vi "fpga_sysID_Z_axis_simple.vi"() -> ()   [LabVIEW 2017]
uses:
  controls/boolean_info.ctl
  sysID_Z-axis-params.ctl
  <vilib>/rvi/Emulation/niFpgaGetClockAttributes.vi
  <vilib>/rvi/Emulation/niFpgaSctlEmulationGetInTimedLoop.vi
  <vilib>/rvi/Emulation/niFpgaEmulationReportErrorSimple.vi
  <vilib>/rvi/Emulation/niFpgaProcessEmulError.vi
  <vilib>/rvi/eio/common/nirviEmuTemplateMethod_errors.vi
  <vilib>/rvi/DataTransferAndStorage/Container/Common/niFpgaContainerExecOnDevCompGetState.vi
  <vilib>/rvi/Emulation/niFpgaEmulationIsFPGAContextNoSignature.vi
  <vilib>/rvi/errors/niFpgaSetErrorForExecOnDevCompSimple.vi
  <vilib>/rvi/eio/common/nirviEmuReportErrorAndStop.vi
  <vilib>/rvi/DataTransferAndStorage/Container/Common/niFpgaContainerGetUniqueNameForEmu.vi
  <vilib>/rvi/FIFO/Fifo_Resource/nirvififoEmulationSetSize.vi
  <vilib>/rvi/FIFO/Fifo_Resource/nirviFifoEmulationQueueMgr.vi
  <instcachedir>/0/nirviFifoEmulationQueueMgr_E5CAEC123FF24DC58D834DCA3CDAA9B5.lvgen/nirviFifoEmulationQueueMgr_E5CAEC123FF24DC58D834DCA3CDAA9B5_006.vi
  <vilib>/rvi/FIFO/Fifo_Resource/nirvififoEmulationDetermineInputValidOut.vi
  <vilib>/rvi/FIFO/Fifo_Resource/nirvififoEmulationCreateLock.vi
  <vilib>/rvi/FIFO/Fifo_Resource/nirvififoEmulationObtainLock.vi
  <vilib>/rvi/FIFO/Fifo_Resource/nirvififoEmulationReleaseLock.vi
  <vilib>/rvi/occurrence/nirviWaitOnOccurrenceBase.vi
  <vilib>/rvi/errors/nirviReportUnexpectedCaseInternalError.vi
  <vilib>/rvi/errors/nirviReportUnexpectedCaseInternalError (U32).vi
  <vilib>/Utility/error.llb/Clear Errors.vi
  <vilib>/rvi/interface/RandomDataEmulation/niFpgaRandomDataHandleErrors.vi
  <vilib>/rvi/Memory/Memory_Emulation/niFpgaMemoryEmulationCacheClearOnFirstRun.vi
  <vilib>/rvi/Memory/Memory_Emulation/nirvimemoryEmulationManagerCache_MakeExclusive.vi
  <vilib>/rvi/Memory/Memory_Emulation/niFpgaMemoryEmulationValidateCache.vi
  <vilib>/rvi/Memory/Memory_Emulation/nirvimemoryEmulationManagerCache_InsertValue.vi
  <vilib>/rvi/Memory/Memory_Emulation/nirvimemoryEmulationManagerCache_ReleaseExclusive.vi
  <vilib>/rvi/Memory/Memory_Emulation/nirvimemoryEmulationManagerCache_GetValue.vi
  <vilib>/rvi/Memory/Memory_Emulation/nirvimemoryEmulationManagerCache_SetValue.vi
  <vilib>/rvi/Emulation/niFpgaCriticalErrorInLSC.vi
  <vilib>/eio/EIONode/EIONode.xnode
  <vilib>/rvi/DataTransferAndStorage/Container/XNode/niFpgaContainer.xnode
  <vilib>/rvi/FIFO/Fifo_Resource/niFpgaFifoEmulationRefIn.vi
  <vilib>/rvi/DataTransferAndStorage/Register/Emulation/niFpgaRegisterEmulation.vi
  libimaging-cs.lvlib
panel:
  out "logging-timeout?":bool
  in  "sysID_Z_axis_params":T1={"TOL"=0.3, "ramp-rate"=-5e-06, "z-u-max"=5.0, "offset"=0.0, "Ki"=0.001, "Z-error-threshold"=0.0, "Z-settled-samples\nthreshold "=0, "z_UP"=1.5, "zup-N"=5000} {"Z-error-threshold" format="%#_13g"; "ramp-rate" format="%#_4g"; "TOL" format="%#_13g"}
  out "iter":i32
  out "All Done":bool
  in  "TsTicks":u32=1600
  out "Current Case":i16
  out "boolean \nindicators":T2
  out "z-u(k)":sgl
  in  "ABORT":bool
  out "read fifo HARD timeout":bool
  out "e(0) (threshhold init)":fxp<+/-,16,5>
  in  "init Z up":fxp<+/-,16,5>
  in  "trigger-0":bool
  in  "initial case":i16
  # "- If collect all = fasle and collect move = false,\nwe only collect measurement data.\n- If collect all = false, and collect move = true,\nwe collect measurement and move data.\n- If collect all = true, we collect everything."
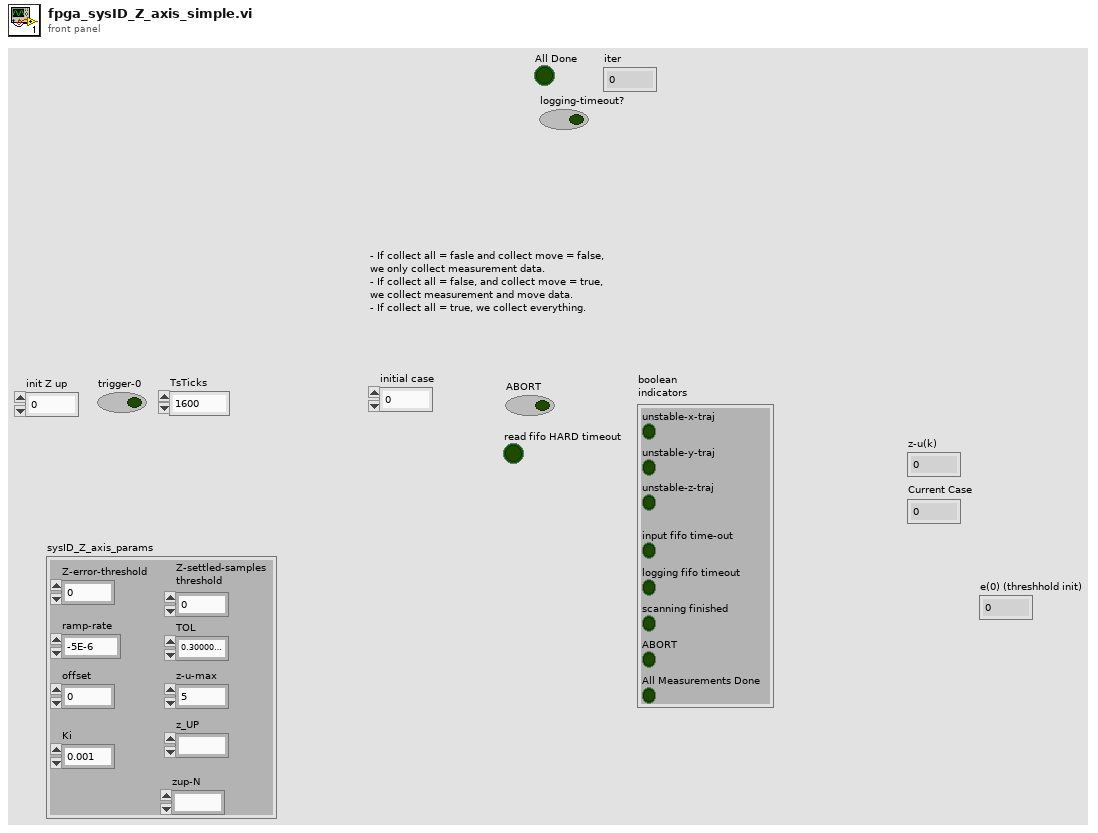
[diagram p1: front panel]
types:
  T1 = typedef "sysID_Z-axis-params.ctl" = cluster{"TOL":sgl, "ramp-rate":sgl, "z-u-max":sgl, "offset":sgl, "Ki":sgl, "Z-error-threshold":sgl, "Z-settled-samples\nthreshold ":i16, "z_UP":fxp<+/-,16,5>, "zup-N":i16}
  T2 = typedef "boolean_info.ctl" = cluster{"unstable-z-traj":bool, "input fifo time-out":bool, "logging fifo timeout":bool, "scanning finished":bool, "unstable-x-traj":bool, "unstable-y-traj":bool, "ABORT":bool, "All Measurements Done":bool}
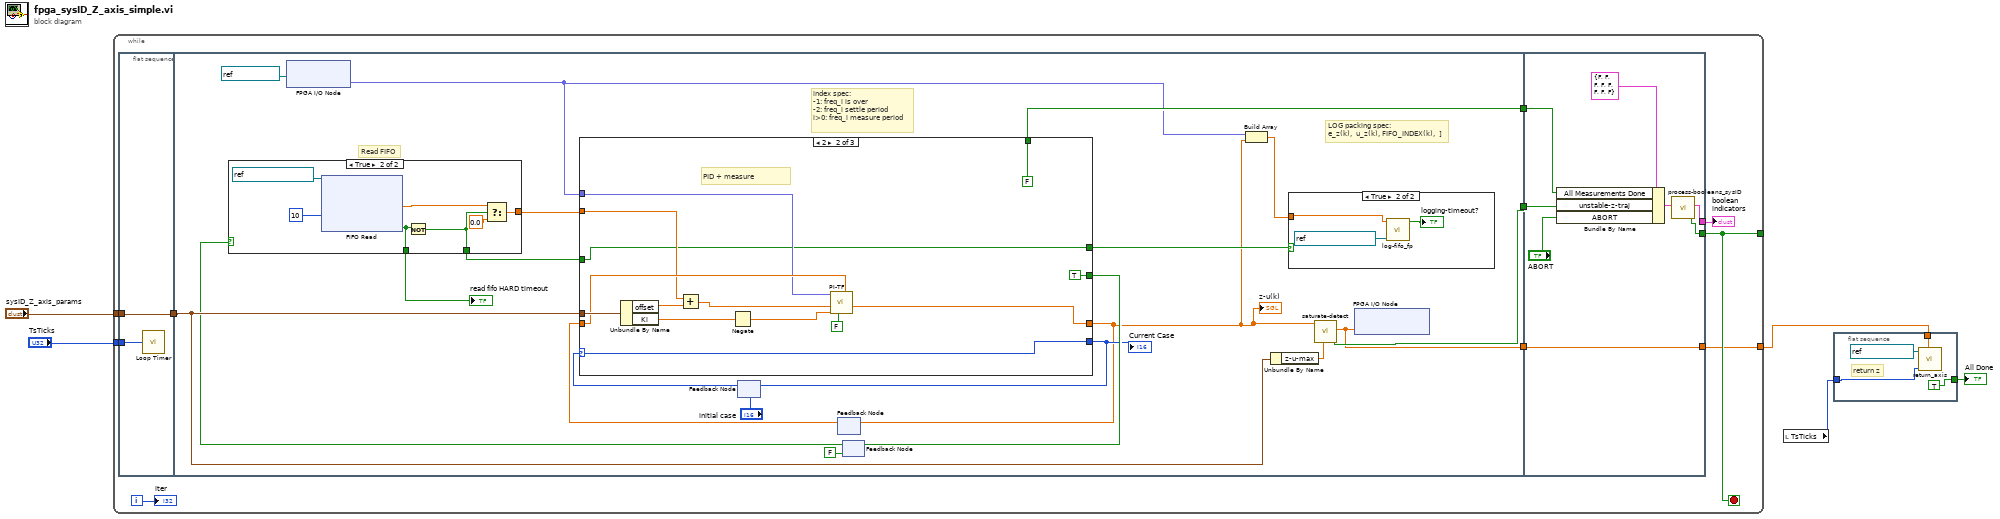
[diagram p0: block diagram]
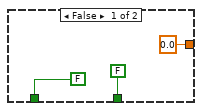
[diagram p3: hidden frame]
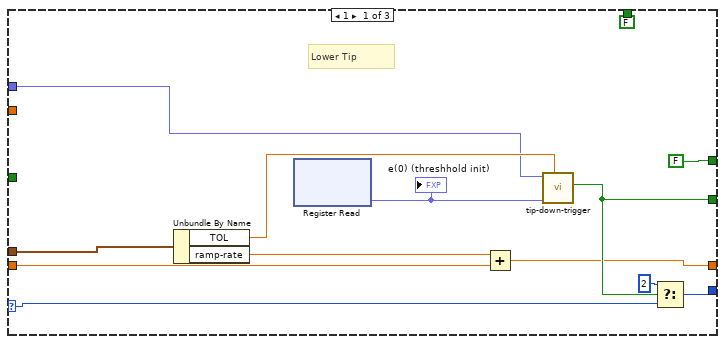
[diagram p4: hidden frame]
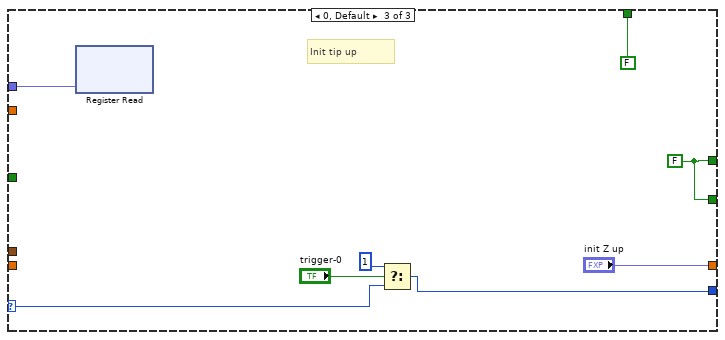
[diagram p5: hidden frame]
diagram:
  n1 = while {
    tunnel: "sysID_Z_axis_params" -> [w12]
    tunnel: "TsTicks" -> [w11]
    tunnel: [w9] -> _
    tunnel: [w7] -> w4
    i -> [w6]
    stop <- w9 stop-if-true
    n2 = flat-sequence {
      tunnel: w11 -> [w16]
      tunnel: w12 -> [w17]
      tunnel: [w17] -> w15
      tunnel: w15 -> [w29]
      tunnel: [w33] -> w14
      tunnel: [w27] -> w13
      tunnel: [w31] -> w8
      tunnel: w14 -> [w93]
      tunnel: w13 -> [w90]
      tunnel: [w86] -> w9
      tunnel: [w87] -> w10
      tunnel: [w89] -> w7
      tunnel: w8 -> [w89]
      frame #0 {
        n3 = call "Loop Timer"("Count(Ticks)"=w16) -> ()  [unwired: 1 out]
      }
      frame #1 {
        # "index spec:\n-1: freq_i is over\n-2: freq_i settle period\ni>0: freq_i measure period"
        # "LOG packing spec:\ne_z(k),  u_z(k), FIFO_INDEX(k),  ]"
        # "Read FIFO"
        n4 = xnode "FPGA I/O Node"("FPGA I/O In"=refnum<k21> "Mod2/AI2" ("y - ADC")) -> ("I/O Item"=w23:fxp<+/-,24,5>)  [unwired: 1 out]
        n5 = feedback #1("initial case") -> (w36:i16)
        n6 = feedback #2() -> (w35:sgl)  [unwired: 1 in]
        n7 = feedback #3(FALSE ("trigger-0")) -> (w18:bool)
        n8 = case shown="True" w18 {
          tunnel: [sgl 0.0 ("Element") w49] -> w30
          tunnel: [FALSE ("Timed Out?") w45] -> w21
          tunnel: [FALSE w44] -> w20
          frame False {
          }
          frame True {
            n9 = xnode ("FIFO Read")("Timeout"=10, "FIFO In"=refnum<k21> "host_to_fpga_fp") -> ("Element"=w46:sgl, "Timed Out?"=w45:bool)  [unwired: 1 out]
            n10 = Not(x=w45) -> (.not. x?=w44:bool)
            n11 = Select(t=w46, s=w44, f=sgl 0.0) -> (s? t:f=w49:sgl)
          }
        }
        "read fifo HARD timeout" <- w21
        n12 = case shown="2" w36 {
          selector: w36 -> [w60 w66 w83]
          tunnel: [FALSE w65 w78] -> w25
          tunnel: [w58 w66 w85] -> w26
          tunnel: w23 -> [w51 w68 w79]
          tunnel: [w53 TRUE ("trigger-0") w78] -> w32
          tunnel: [w52 w72 "init Z up"] -> w22
          tunnel: w35 -> [w56 w73 _]
          tunnel: w29 -> [w59 w74 _]
          tunnel: w30 -> [_ w67 _]
          tunnel: [FALSE FALSE FALSE] -> w27
          tunnel: w20 -> [_ w65 _]
          frame 1 {
            # "Lower Tip"
            n13 = Unbundle By Name(w59) -> ("TOL"=w62:sgl, "ramp-rate"=w61:sgl)
            n14 = xnode ("Register Read")() -> ("Data"=w63:fxp<+/-,16,5>)  [unwired: 1 in, 1 out]
            "e(0) (threshhold init)" <- w63
            n15 = Add(x=w61, y=w56) -> (x+y=w52:sgl)
            n16 = call "tip-down-trigger.vi"("TOL"=w62, "Vo"=w63, "e(k)"=w51) -> ("trigger"=w53:bool)  [unwired: 8 in]
            n17 = Select(t=i16 2, s=w53, f=w60) -> (s? t:f=w58:i16)
          }
          frame 2 {
            # "PID + measure"
            n18 = Unbundle By Name(w74) -> ("offset"=w70:sgl, "Ki"=w75:sgl)
            n19 = Add(x=w67, y=w70) -> (x+y=w71:sgl)
            n20 = Negate(x=w75) -> (-x=w76:sgl)
            n21 = call "PI-TF.vi"("u(k-1)"=w73, "reset"=FALSE, "Ki"=w76, "setpoint"=w71, "y(k)"=w68) -> ("u(k)"=w72:sgl)  [unwired: 6 in]
          }
          frame 0, Default {
            w78 = FALSE
            # "Init tip up"
            n22 = xnode ("Register Read")("Data"=w79) -> ()  [unwired: 1 in, 1 out]
            n23 = Select(t=i16 1, s="trigger-0", f=w83) -> (s? t:f=w85:i16)
          }
        }
        "z-u(k)" <- w22
        "Current Case" <- w26
        n24 = feedback-in #1(w26) -> ()
        n25 = feedback-in #2(w22) -> ()
        n26 = feedback-in #3(w32) -> ()
        n27 = Build Array(w23, w22) -> (w34:sgl[])
        n28 = Unbundle By Name(w29) -> ("z-u-max"=w28:sgl)
        n29 = case shown="True" w25 {
          tunnel: w34 -> [_ w40]
          frame False {
          }
          frame True {
            n30 = call "log-fifo_fp.vi"("FIFO In"=refnum<k21> "fpga_to_host_fp", "input-data"=w40) -> ("logging-timeout?"=→"logging-timeout?":bool)  [unwired: 9 in]
          }
        }
        n31 = call "saturate-detect.vi"("bound"=w28, "x"=w22) -> ("saturated"=w33:bool, "sat(x)"=w31:sgl)  [unwired: 8 in]
        n32 = xnode "FPGA I/O Node"("Mod1/AO2"=w31) -> ()  [unwired: 1 in, 1 out]
      }
      frame #2 {
        n33 = Bundle By Name(cluster=T2 {"unstable-z-traj"=FALSE, "input fifo time-out"=FALSE, "logging fifo timeout"=FALSE, "scanning finished"=FALSE, "unstable-x-traj"=FALSE, "unstable-y-traj"=FALSE, "ABORT"=FALSE, "All Measurements Done"=FALSE} ("boolean errors"), "All Measurements Done"=w90, "unstable-z-traj"=w93, "ABORT"="ABORT") -> (w88:T2)
        n34 = call "process-booleans_sysID.vi"("boolean indicators 2"=w88) -> ("scaning finished"=w86:bool, "boolean indicators"=w87:T2)  [unwired: 9 in]
      }
    }
    "boolean \nindicators" <- w10
    "iter" <- w6
  }
  n35 = local read "TsTicks"() -> (w1:u32)
  n36 = flat-sequence {
    tunnel: w4 -> [w97]
    tunnel: [TRUE] -> w3
    tunnel: w1 -> [w94]
    frame #0 {
      # "return z"
      n37 = call "return_axis.vi"("u(0)"=w97, "TsTicks"=w94, "FPGA I/O In"=refnum<k21> "Mod1/AO2") -> ()  [unwired: 9 in]
    }
  }
  "All Done" <- w3
